vi "OrderBook-Test-1.vi"() -> ()   [LabVIEW 2016]
uses:
  Host-Command-for-Fpga.ctl
panel:
  out "Sorted Order Book":string[](array[string])
  in  "Ticker":string="AAPL"
  out "RawResults":u64[](array[numeric]) format="%.0x"
  in  "error in":errorcluster
  out "Command":u64[](array[numeric]) format="%.0x"
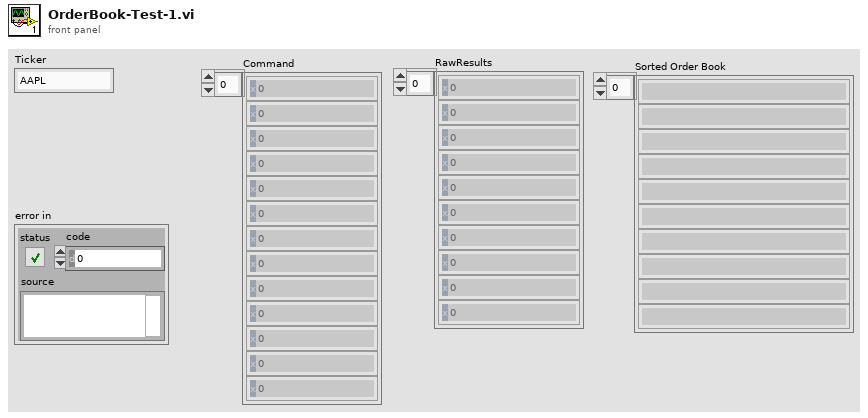
[diagram p1: front panel]
types:
  T1 = typedef "Host-Command-for-Fpga.ctl" = cluster{"Side":enum16{"Buy", "Sell"}, "Operation":enum16{"GetAll", "AddOrder", "DeleteOrder"}, "Price":dbl, "# of Shares":u32, "OrderRefNum":u64}
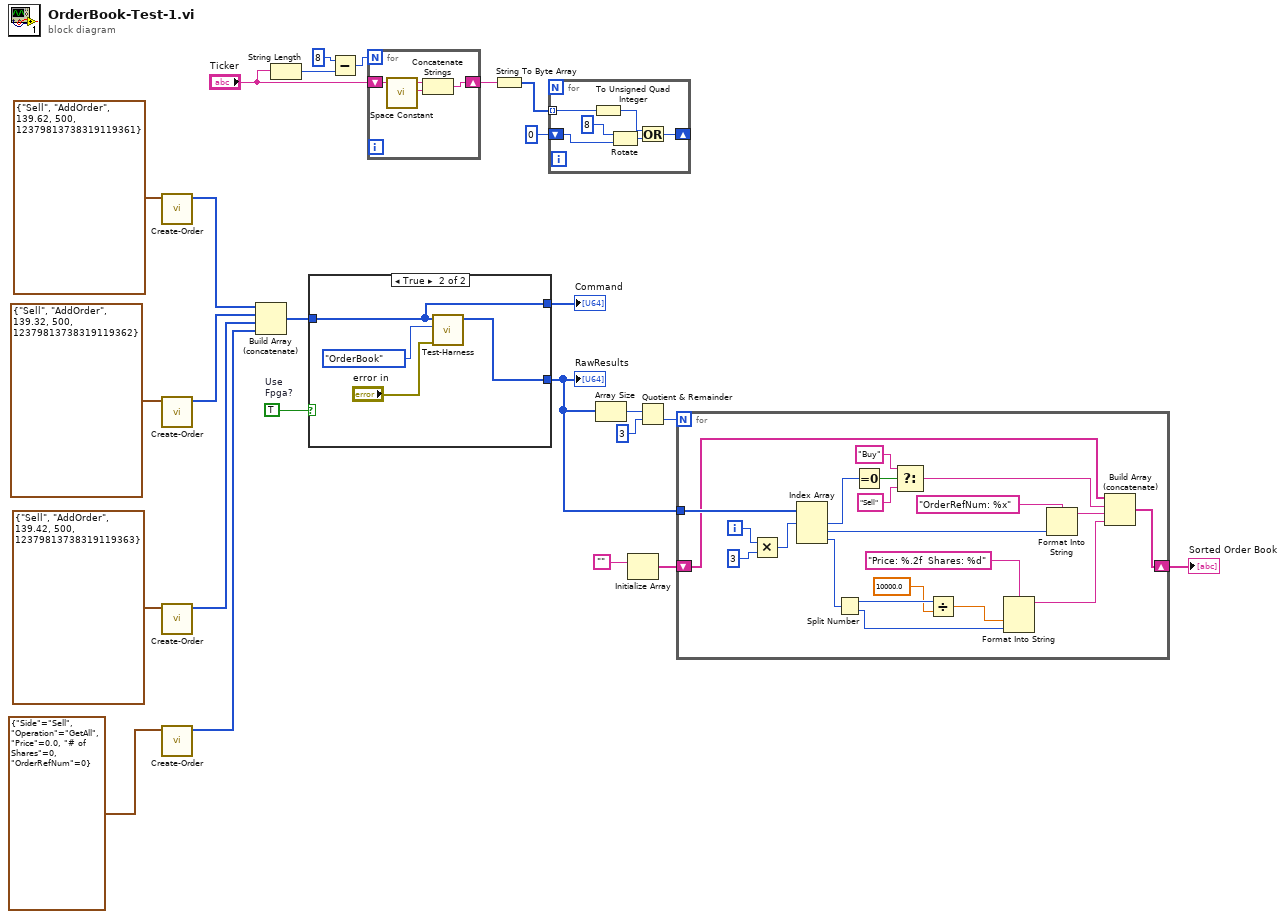
[diagram p0: block diagram]
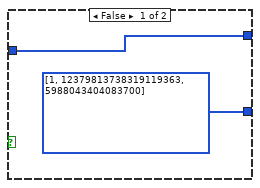
[diagram p2: hidden frame]
diagram:
  w18 = TRUE  # Use Fpga?
  n1 = call "Create-Order.vi"("Command"=T1 {"Side"=enum."Sell", "Operation"=enum."AddOrder", "Price"=139.62, "# of Shares"=500, "OrderRefNum"=12379813738319119361}) -> ("Array"=w17:u64[])  [unwired: 10 in]
  n2 = call "Create-Order.vi"("Command"=T1 {"Side"=enum."Sell", "Operation"=enum."AddOrder", "Price"=139.32, "# of Shares"=500, "OrderRefNum"=12379813738319119362}) -> ("Array"=w16:u64[])  [unwired: 10 in]
  n3 = call "Create-Order.vi"("Command"=T1 {"Side"=enum."Sell", "Operation"=enum."AddOrder", "Price"=139.42, "# of Shares"=500, "OrderRefNum"=12379813738319119363}) -> ("Array"=w13:u64[])  [unwired: 10 in]
  n4 = call "Create-Order.vi"("Command"=T1 {"Side"=enum."Sell", "Operation"=enum."GetAll", "Price"=0.0, "# of Shares"=0, "OrderRefNum"=0}) -> ("Array"=w12:u64[])  [unwired: 10 in]
  n5 = Build Array (concatenate)(w17, w16, w13, w12) -> (w15:u64[])
  n6 = String Length(string="Ticker") -> (length=w25:i32)
  n7 = case shown="True" w18 {
    tunnel: w15 -> [w27 w29]
    tunnel: [w27 w29] -> w14
    tunnel: [u64[] [1, 12379813738319119363, 5988043404083700] ("DataOut") w28] -> w4
    frame False {
    }
    frame True {
      n8 = call "Test-Harness.vi"("error in"="error in", "Operating\nMode"=enum16{"OrderBook"}."OrderBook" ("Operating\nMode"), "DataIn"=w29) -> ("DataOut"=w28:u64[])  [unwired: 7 in, 1 out]
    }
  }
  "Command" <- w14
  "RawResults" <- w4
  n9 = Subtract(x=8, y=w25) -> (x-y=w23:i32)
  n10 = for {
    N: w23 -> [_]
    shift-right: [w32] -> w21
    shift-left: "Ticker" -> [w34]
    n11 = call <vilib>:"Space Constant.vi"() -> ("String"=w33:string)
    n12 = Concatenate Strings(w34, w33) -> (w32:string)
  }
  n13 = String To Byte Array(string=w21) -> (unsigned byte array=w19:u8[])
  n14 = for {
    shift-right: [w38] -> _
    shift-left: u64 0 -> [w36]
    tunnel: w19 -> [w40] mode=indexing
    n15 = To Unsigned Quad Integer(1:w40) -> (0:w37:u64)
    n16 = Rotate(1:w36, 2:i16 8 ("y")) -> (0:w39:u64)
    n17 = Or(x=w37, y=w39) -> (x .or. y?=w38:u64)
  }
  n18 = Array Size(array=w4) -> (size(s)=w7:i32)
  n19 = Initialize Array("") -> (w2:string[])  [unwired: 1 in]
  n20 = Quotient & Remainder(x=w7, y=3) -> (floor(x/y)=w5:i32)  [unwired: 1 out]
  n21 = for {
    N: w5 -> [_]
    tunnel: w4 -> [w61]
    shift-right: [w41] -> w1
    shift-left: w2 -> [w42]
    i -> [w59]
    n22 = Multiply(x=w59, y=3) -> (x*y=w60:i32)
    n23 = Index Array(array=w61, index #1=w60) -> (element #1=w50:u64, element #2=w57:u64, element #3=w54:u64)  [unwired: 2 in]
    n24 = Split Number(x=w54) -> (hi(x)=w45:u32, lo(x)=w53:u32)
    n25 = Equal To 0?(x=w50) -> (x = 0?=w49:bool)
    n26 = Select(t="Buy", s=w49, f="Sell") -> (s? t:f=w46:string)
    n27 = Divide(x=w45, y=10000.0) -> (x/y=w43:dbl)
    n28 = Format Into String(format string="Price: %.2f  Shares: %d", w43, w53) -> (resulting string=w51:string)  [unwired: 2 in, 1 out]
    n29 = Format Into String(format string="OrderRefNum: %x" ("initial string"), w57) -> (resulting string=w56:string)  [unwired: 2 in, 1 out]
    n30 = Build Array (concatenate)(w42, w46, w56, w51) -> (w41:string[])
  }
  "Sorted Order Book" <- w1
